vi "Is Embedded Data Logger Custom Device Enabled.vi"(8 "error in":errorcluster, 11 "embedded data logger in":T1 format="%.0x") -> (0 "error out":errorcluster, 2 "enabled":bool, 3 "embedded data logger out":T1 format="%.0x")   [LabVIEW 2027, in "Embedded Data Logger Scripting.lvlib"]
uses:
  Embedded Data Logger Scripting.lvlib
  <vilib>/NI VeriStand/Custom Device API/Custom Device Item Ref.ctl
  Shared/Constants.vi
  Shared/Embedded Data Logger Shared.lvlib
  <vilib>/NI VeriStand/Custom Device API/Custom Device API.lvlib
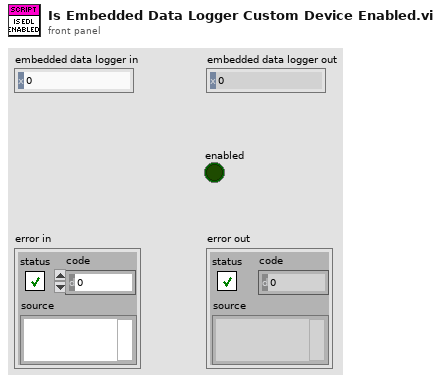
[diagram p1: front panel]
types:
  T1 = typedef "Custom Device API.lvlib/Custom Device Item Ref.ctl" = u64
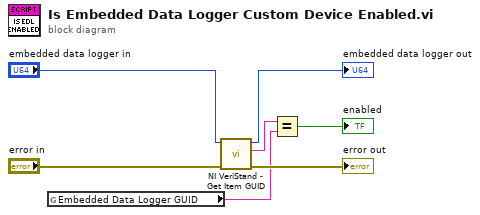
[diagram p0: block diagram]
diagram:
  n1 = global read "Constants.vi" "Embedded Data Logger GUID"() -> (w1:string)
  n2 = call <vilib>:"NI VeriStand - Get Item GUID.vi"("error in (no error)"="error in", "Item Ref in"="embedded data logger in") -> ("error out"=→"error out":errorcluster, "GUID"=w2:string, "Item Ref out"=→"embedded data logger out":T1)  [unwired: 7 in]
  n3 = Equal?(x=w2, y=w1) -> (x = y?=→"enabled":bool)
